vi "AutoBalance.vi"(8 "error in (no error)":errorcluster) -> (0 "error out":errorcluster)   [LabVIEW 2020]
doc: "Wrapper class for drive straight"
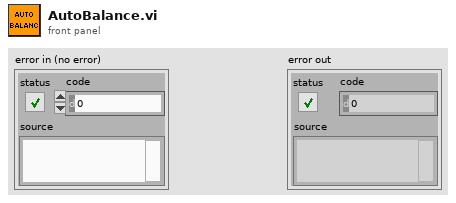
[diagram p1: front panel]
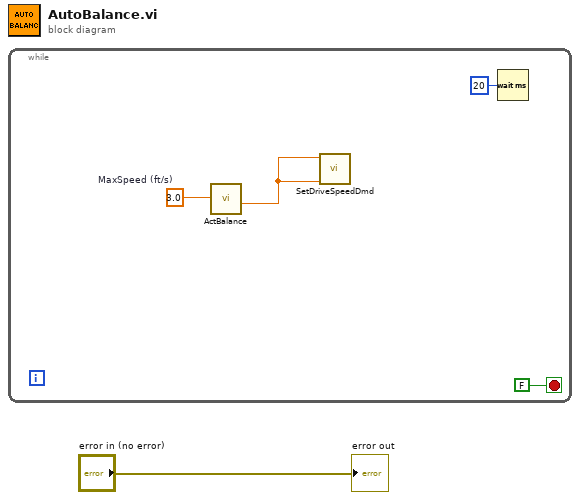
[diagram p0: block diagram]
diagram:
  n1 = while {
    stop <- FALSE stop-if-true
    w3 = 3.0  # MaxSpeed (ft/s)
    n2 = call "ActBalance.vi"("MaxSpeed (ft/s)"=w3) -> ("XSpeedDemand"=w2:dbl)  [unwired: 9 in, 1 out]
    n3 = call "SetDriveSpeedDmd.vi"("LeftSpeedInput"=w2, "RightSpeedInput"=w2) -> ()  [unwired: 10 in]
    n4 = Wait (ms)(milliseconds to wait=u32 20) -> ()  [unwired: 1 out]
  }
  "error out" <- "error in (no error)"
